vi "ProdaNG.DebugLogger.vi"(6 "return type":i32, 7 "cmd":string, 8 "error in (no error)":errorcluster, 11 "done? (F)":bool) -> (0 "error out":errorcluster)   [LabVIEW 2016]
uses:
  ProdaNG.Global.vi
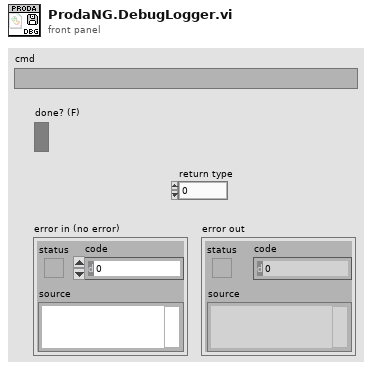
[diagram p1: front panel]
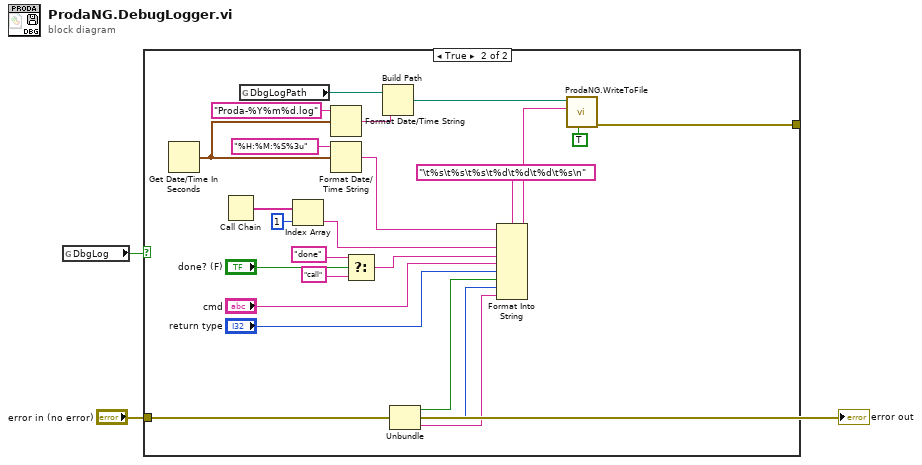
[diagram p0: block diagram]
diagram:
  n1 = global read "ProdaNG.Global.vi" "DbgLog"() -> (w1:bool)
  n2 = case shown="True" w1 {
    tunnel: "error in (no error)" -> [_ w12]
    tunnel: [_ w3] -> _
    frame False {
    }
    frame True {
      n3 = Get Date/Time In Seconds() -> (seconds since 1Jan1904=w23:timestamp)
      n4 = Call Chain() -> (call chain=w19:string[])
      n5 = global read "ProdaNG.Global.vi" "DbgLogPath"() -> (w7:path)
      n6 = Index Array(array=w19, index=1) -> (element=w18:string)
      n7 = Format Date/Time String(time format string (%c)="Proda-%Y%m%d.log", seconds (now)=w23) -> (date/time string=w25:string)  [unwired: 1 in]
      n8 = Format Date/Time String(time format string (%c)="%H:%M:%S%3u", seconds (now)=w23) -> (date/time string=w21:string)  [unwired: 1 in]
      n9 = Select(t="done" ("format string"), s="done? (F)", f="call" ("format string")) -> (s? t:f=w15:string)
      n10 = Build Path(base path=w7, name or relative path=w25) -> (appended path=w5:path)
      n11 = Unbundle(w12) -> ("status"=w11:bool, "code"=w10:i32, "source"=w9:string)
      n12 = Format Into String(format string="\t%s\t%s\t%s\t%d\t%d\t%d\t%s\n", initial string=w21, w18, w15, "cmd", "return type", w11, w10, w9) -> (resulting string=w6:string)  [unwired: 1 in, 1 out]
      n13 = call "ProdaNG.WriteToFile.vi"("append (F)"=TRUE, "addition"=w6, "file"=w5) -> ("error out"=w3:errorcluster)  [unwired: 8 in]
    }
  }
  "error out" <- "error in (no error)"
